vi "Get.vi"(11 "ID in":refnum<class "ID.lvclass">) -> (2 "Entity ID":T1)   [LabVIEW 2020, in "Conditu2.lvlib" / "Columns.lvlib" / "ID.lvclass"]
uses:
  ID.lvclass
  Entity ID.ctl
  ID.lvclass/ID.ctl
  Conditu2.lvlib
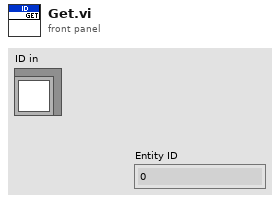
[diagram p1: front panel]
types:
  T1 = typedef "Conditu2.lvlib/Entity ID.ctl" = i64
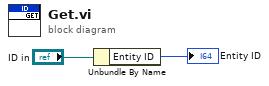
[diagram p0: block diagram]
diagram:
  n1 = Unbundle By Name("ID in") -> ("Entity ID"=→"Entity ID":T1)
